vi "usbos.vi"() -> ()   [LabVIEW 2025]
uses:
  <vilib>/Instr/_visa.llb/VISA Configure Serial Port (Instr).vi
panel:
  out "XY Graph":cluster{dbl[], dbl[]}(graph)
  out "error out":errorcluster
  in  "interval":i16
  in  "fire":bool
  out "read buffer":string
  in  "stop":bool
  # "1."
  # "2."
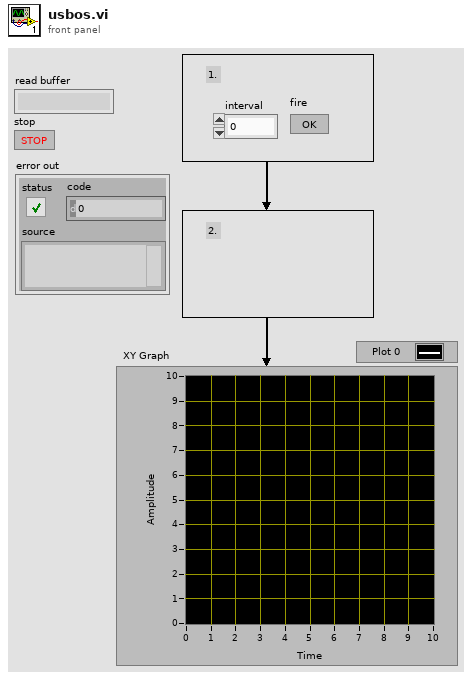
[diagram p1: front panel]
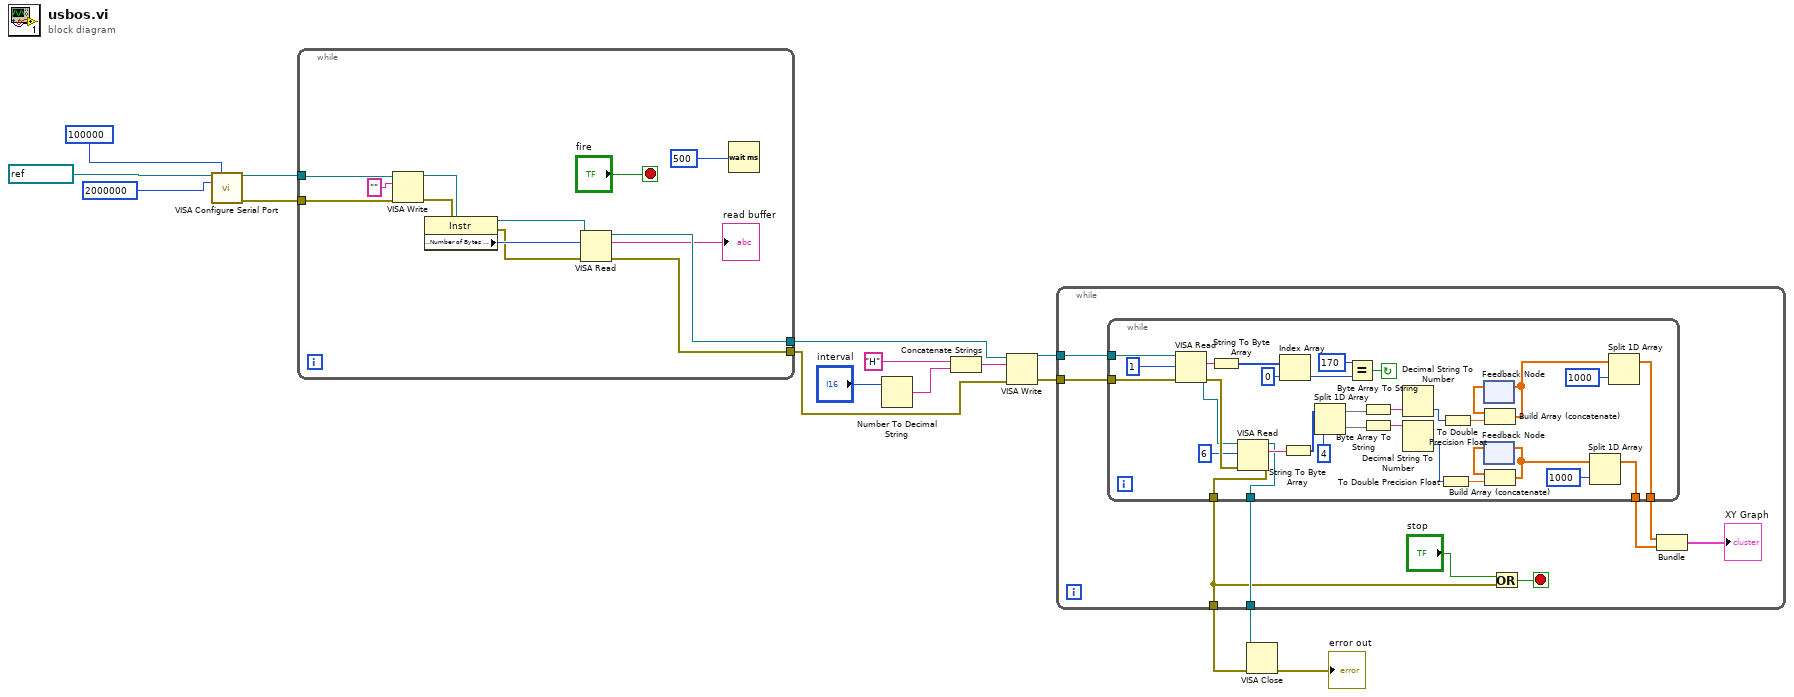
[diagram p0: block diagram]
diagram:
  n1 = call-poly "VISA Configure Serial Port"("VISA resource name"=refnum<visa-resource-name> "COM6", "timeout (10sec)"=u32 100000, "baud rate (9600)"=u32 2000000) -> ("VISA resource name out"=w14:refnum<visa-resource-name>, "error out"=w13:errorcluster)  [unwired: 11 in]
  n2 = while {
    tunnel: w14 -> [w19]
    tunnel: w13 -> [w21]
    tunnel: [w20] -> w7
    tunnel: [w25] -> w6
    stop <- "fire" stop-if-true
    n3 = VISA Write(VISA resource name=w19, write buffer="", error in (no error)=w21) -> (VISA resource name out=w29:refnum<visa-resource-name>, error out=w28:errorcluster)  [unwired: 1 out]
    n4 = property class="Instr"(reference=w29, error in=w28) -> (reference out=w27:refnum<visa-resource-name>, error out=w18:errorcluster, "Serial Settings:Number of Bytes at Serial Port"=w26:u32)
    n5 = VISA Read(VISA resource name=w27, byte count=w26, error in (no error)=w18) -> (VISA resource name out=w25:refnum<visa-resource-name>, read buffer=→"read buffer":string, error out=w20:errorcluster)  [unwired: 1 out]
    n6 = Wait (ms)(milliseconds to wait=u32 500 ("millisecond timer value")) -> ()  [unwired: 1 out]
  }
  n7 = Number To Decimal String(number="interval") -> (decimal integer string=w10:string)  [unwired: 1 in]
  n8 = Concatenate Strings("H", w10) -> (w8:string)
  n9 = VISA Write(VISA resource name=w6, write buffer=w8, error in (no error)=w7) -> (VISA resource name out=w4:refnum<visa-resource-name>, error out=w5:errorcluster)  [unwired: 1 out]
  n10 = while {
    tunnel: w5 -> [w38]
    tunnel: w4 -> [w37]
    tunnel: [w31] -> w2
    tunnel: [w32] -> w1
    stop <- w30 stop-if-true
    n11 = while {
      tunnel: w38 -> [w67]
      tunnel: w37 -> [w65]
      tunnel: [w48] -> w35
      tunnel: [w47] -> w34
      tunnel: [w45] -> w31
      tunnel: [w39] -> w32
      stop <- w59 continue-if-true
      n12 = VISA Read(VISA resource name=w65, byte count=u32 1, error in (no error)=w67) -> (VISA resource name out=w40:refnum<visa-resource-name>, read buffer=w70:string, error out=w46:errorcluster)  [unwired: 1 out]
      n13 = String To Byte Array(string=w70) -> (unsigned byte array=w41:u8[])
      n14 = VISA Read(VISA resource name=w40, byte count=u32 6, error in (no error)=w46) -> (VISA resource name out=w39:refnum<visa-resource-name>, read buffer=w44:string, error out=w45:errorcluster)  [unwired: 1 out]
      n15 = Index Array(array=w41, index=0) -> (element=w71:u8)
      n16 = String To Byte Array(string=w44) -> (unsigned byte array=w42:u8[])
      n17 = Split 1D Array(array=w42, index=4) -> (first subarray=w63:u8[], second subarray=w62:u8[])
      n18 = Equal?(x=u8 170, y=w71) -> (x = y?=w59:bool)
      n19 = Byte Array To String(unsigned byte array=w63) -> (string=w61:string)
      n20 = Byte Array To String(unsigned byte array=w62) -> (string=w60:string)
      n21 = Decimal String To Number(string=w61) -> (number=w54:i32)  [unwired: 2 in, 1 out]
      n22 = Decimal String To Number(string=w60) -> (number=w53:i32)  [unwired: 2 in, 1 out]
      n23 = To Double Precision Float(number=w53) -> (double precision float=w56:dbl)
      n24 = To Double Precision Float(number=w54) -> (double precision float=w55:dbl)
      n25 = feedback #1() -> (w58:dbl[])  [unwired: 1 in]
      n26 = feedback #2() -> (w57:dbl[])  [unwired: 1 in]
      n27 = Build Array (concatenate)(w58, w55) -> (w52:dbl[])
      n28 = feedback-in #1(w52) -> ()
      n29 = Build Array (concatenate)(w57, w56) -> (w49:dbl[])
      n30 = feedback-in #2(w49) -> ()
      n31 = Split 1D Array(array=w49, index=1000) -> (first subarray=w47:dbl[])  [unwired: 1 out]
      n32 = Split 1D Array(array=w52, index=1000) -> (first subarray=w48:dbl[])  [unwired: 1 out]
    }
    n33 = Or(x="stop", y=w31) -> (x .or. y?=w30:bool)
    n34 = Bundle(w35, w34) -> (→"XY Graph":cluster{dbl[], dbl[]})  [unwired: 1 in]
  }
  n35 = VISA Close(VISA resource name=w1, error in (no error)=w2) -> (error out=→"error out":errorcluster)
